vi "Write.vi"(8 "error in (no error)":errorcluster, 10 "Data to Write":string, 11 "TCP Connection in":refnum<class "TCP Connection.lvclass">) -> (0 "error out":errorcluster, 3 "TCP Connection out":refnum<class "TCP Connection.lvclass">)   [LabVIEW 2020, in "TCP Connection.lvclass"]
uses:
  <vilib>/gpm_packages/@cs/Network-interface/Source/TCP Interface/TCP Connection/TCP Connection.lvclass
  <vilib>/gpm_packages/@cs/Network-interface/Source/TCP Interface/TCP Connection/TCP Connection.lvclass/TCP Connection.ctl
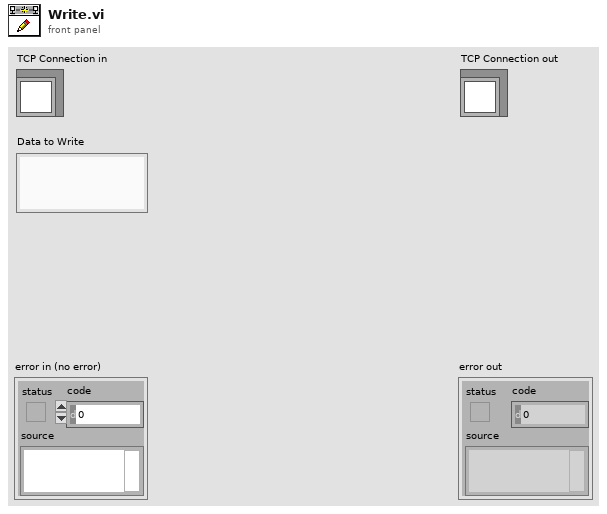
[diagram p1: front panel]
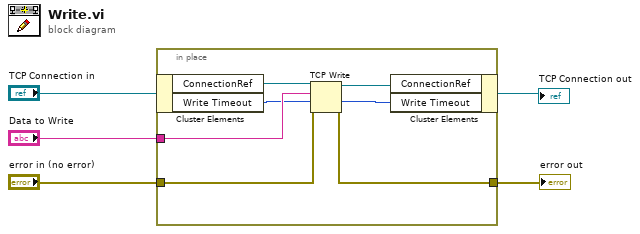
[diagram p0: block diagram]
diagram:
  n1 = in-place {
    in-place-border: "Data to Write" -> [w10]
    in-place-border: "error in (no error)" -> [w9]
    in-place-border: [w6] -> w2
    n2 = in-place-cluster #1("TCP Connection in") -> ("ConnectionRef"=w11:refnum<k5>, "Write Timeout"=w7:i32)
    n3 = TCP Write(connection ID=w11, data in=w10, error in (no error)=w9, 9:w7) -> (connection ID out=w8:refnum<k5>, error out=w6:errorcluster)  [unwired: 1 out]
    n4 = in-place-cluster #1("ConnectionRef"=w8, "Write Timeout"=w7) -> (→"TCP Connection out":refnum<class "TCP Connection.lvclass">)
  }
  "error out" <- w2
